vi "9601 Index not found--error.vi"(8 "error in":errorcluster, 11 "Index":u16) -> (0 "error out":errorcluster)   [LabVIEW 2024]
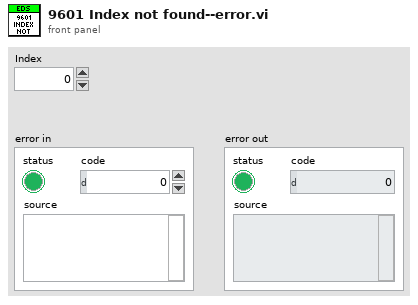
[diagram p1: front panel]
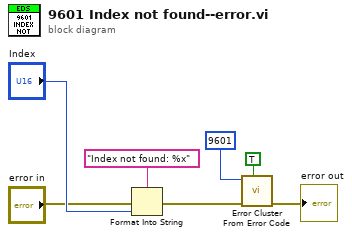
[diagram p0: block diagram]
diagram:
  n1 = Format Into String(format string="Index not found: %x" ("error message (\"\")"), error in="error in", "Index") -> (error out=w5:errorcluster)  [unwired: 1 in, 1 out]
  n2 = call <vilib>:"Error Cluster From Error Code.vi"("show call chain? (False)"=TRUE, "error in (no error)"=w5, "error code (0)"=9601) -> ("error out"=→"error out":errorcluster)  [unwired: 6 in]
